vi "G5.Rest Battery Control.vi"(7 "Functions":T2, 8 "error in":errorcluster, 10 "BatteryControl_Data out":T1, 11 "G5 WEB API in":refnum<class "REST Client.lvclass">) -> (0 "error out":errorcluster, 2 "BatteryControl_Data":T1, 3 "G5 WEB API out":refnum<class "REST Client.lvclass">)   [LabVIEW 2021, in "Regatron.G5.Rest.lvlib"]
doc: "Enables using Battery Control part of G5.REST API\n- Read Energy Count\n- Read Charge Count\n- Reset Counters"
uses:
  Regatron.G5.Rest.lvlib
  <vilib>/addons/_JKI.lib/REST Client/classes/REST Client/REST Client.lvclass
  G5.Rest Battery Control Values.ctl
  G5.Rest Battery Control Functions.ctl
  Regatron.G5.Rest Handle.llb/G5.Rest JsonDB.ctl
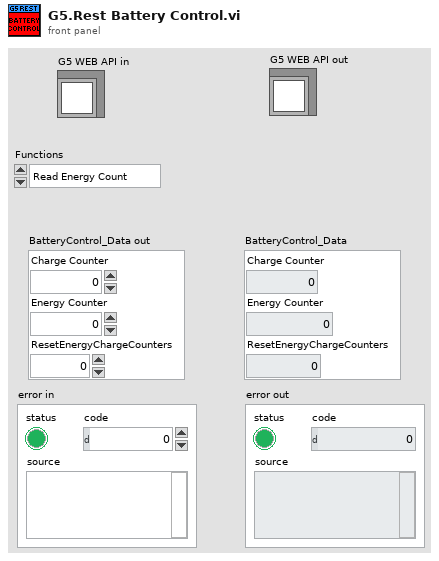
[diagram p1: front panel]
types:
  T1 = typedef "Regatron.G5.Rest.lvlib/G5.Rest Battery Control Values.ctl" = cluster{"Charge Counter":dbl, "Energy Counter":dbl, "ResetEnergyChargeCounters":dbl}
  T2 = typedef "Regatron.G5.Rest.lvlib/G5.Rest Battery Control Functions.ctl" = enum16{"Read Energy Count", "Read Charge Count", "Reset Energy Charge Counters"}
  T3 = typedef "Regatron.G5.Rest.lvlib/G5.Rest JsonDB.ctl" = cluster{"result":dbl}
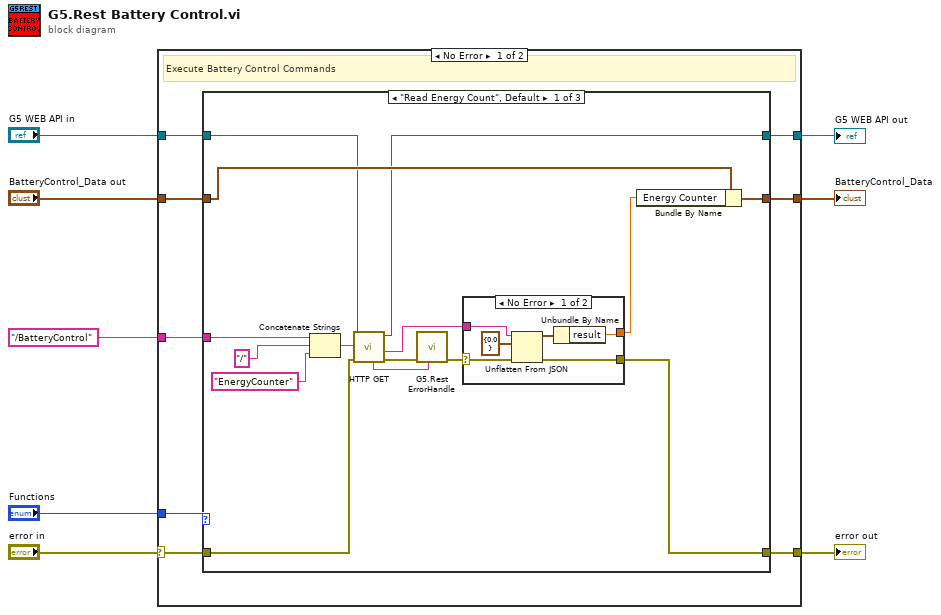
[diagram p0: block diagram]
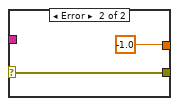
[diagram p2: hidden frame]
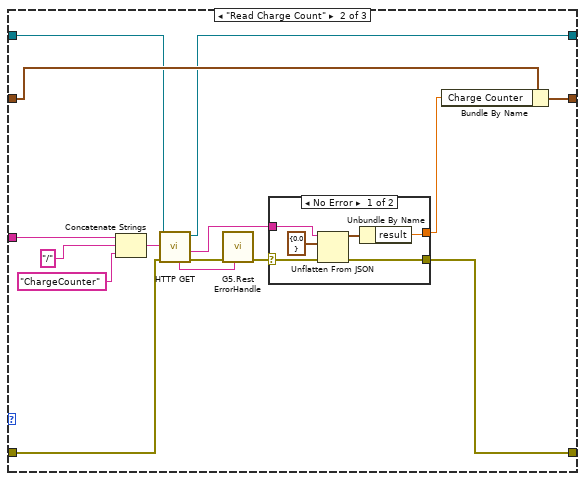
[diagram p3: hidden frame]
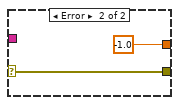
[diagram p4: hidden frame]
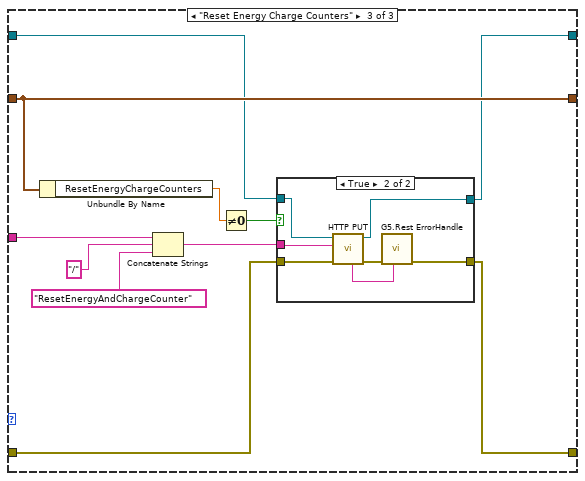
[diagram p5: hidden frame]
diagram:
  n1 = case shown="No Error" "error in" {
    selector: "error in" -> [w12 w83]
    tunnel: [w9 w85] -> w7
    tunnel: "G5 WEB API in" -> [w13 w85]
    tunnel: [w14 w84] -> w5
    tunnel: "BatteryControl_Data out" -> [w15 w84]
    tunnel: "Functions" -> [w16 _]
    tunnel: [w11 w83] -> w2
    tunnel: "/BatteryControl" ("Path") -> [w10 _]
    frame No Error {
      # "Execute Battery Control Commands"
      n2 = case shown="\"Read Energy Count\", Default" w16 {
        tunnel: w15 -> [w31 w54 w69]
        tunnel: [w30 w53 w69] -> w14
        tunnel: w13 -> [w20 w44 w65]
        tunnel: w12 -> [w17 w41 w67]
        tunnel: [w22 w46 w66] -> w11
        tunnel: w10 -> [w28 w52 w71]
        tunnel: [w18 w42 w63] -> w9
        frame "Read Energy Count", Default {
          n3 = Concatenate Strings(w28, "/" ("string"), "EnergyCounter" ("Path")) -> (w19:string)
          n4 = call-dynamic "HTTP GET.vi"("error in (no error)"=w17, "Path"=w19, "REST Client in"=w20) -> ("error out"=w25:errorcluster, "Response body"=w26:string, "REST Client out"=w18:refnum<class "REST Client.lvclass">, "Status String"=w23:string)  [unwired: 3 in, 2 out]
          n5 = call "G5.Rest ErrorHandle.vi"("Status"=w23, "error in (no error)"=w25) -> ("error out"=w24:errorcluster)  [unwired: 9 in]
          n6 = case shown="No Error" w24 {
            selector: w24 -> [w34 w39]
            tunnel: [w37 w39] -> w22
            tunnel: w26 -> [w35 _]
            tunnel: [w32 -1.0 ("result")] -> w21
            frame No Error {
              n7 = Unflatten From JSON(JSON string=w35, type and defaults=T3 {"result"=0.0} ("G5"), error in (no error)=w34) -> (value=w36:T3, error out=w37:errorcluster)  [unwired: 4 in]
              n8 = Unbundle By Name(w36) -> ("result"=w32:dbl)
            }
            frame Error {
            }
          }
          n9 = Bundle By Name(cluster=w31, "Energy Counter"=w21) -> (w30:T1)
        }
        frame "Read Charge Count" {
          n10 = Concatenate Strings(w52, "/" ("string"), "ChargeCounter" ("Path")) -> (w43:string)
          n11 = call-dynamic "HTTP GET.vi"("error in (no error)"=w41, "Path"=w43, "REST Client in"=w44) -> ("error out"=w49:errorcluster, "Response body"=w50:string, "REST Client out"=w42:refnum<class "REST Client.lvclass">, "Status String"=w47:string)  [unwired: 3 in, 2 out]
          n12 = call "G5.Rest ErrorHandle.vi"("Status"=w47, "error in (no error)"=w49) -> ("error out"=w48:errorcluster)  [unwired: 9 in]
          n13 = case shown="No Error" w48 {
            selector: w48 -> [w57 w62]
            tunnel: [w60 w62] -> w46
            tunnel: w50 -> [w58 _]
            tunnel: [w55 -1.0 ("result")] -> w45
            frame No Error {
              n14 = Unflatten From JSON(JSON string=w58, type and defaults=T3 {"result"=0.0} ("G5"), error in (no error)=w57) -> (value=w59:T3, error out=w60:errorcluster)  [unwired: 4 in]
              n15 = Unbundle By Name(w59) -> ("result"=w55:dbl)
            }
            frame Error {
            }
          }
          n16 = Bundle By Name(cluster=w54, "Charge Counter"=w45) -> (w53:T1)
        }
        frame "Reset Energy Charge Counters" {
          n17 = Unbundle By Name(w69) -> ("ResetEnergyChargeCounters"=w73:dbl)
          n18 = Concatenate Strings(w71, "/" ("string"), "ResetEnergyAndChargeCounter" ("Path")) -> (w68:string)
          n19 = Not Equal To 0?(x=w73) -> (x != 0?=w64:bool)
          n20 = case shown="True" w64 {
            tunnel: w68 -> [_ w80]
            tunnel: w67 -> [w75 w79]
            tunnel: [w75 w78] -> w66
            tunnel: w65 -> [w74 w77]
            tunnel: [w74 w76] -> w63
            frame False {
            }
            frame True {
              n21 = call-dynamic "HTTP PUT.vi"("error in (no error)"=w79, "Path"=w80, "REST Client in"=w77) -> ("error out"=w82:errorcluster, "REST Client out"=w76:refnum<class "REST Client.lvclass">, "Status String"=w81:string)  [unwired: 3 in, 3 out]
              n22 = call "G5.Rest ErrorHandle.vi"("Status"=w81, "error in (no error)"=w82) -> ("error out"=w78:errorcluster)  [unwired: 9 in]
            }
          }
        }
      }
    }
    frame Error {
      # "Pass input data in case of error"
    }
  }
  "G5 WEB API out" <- w7
  "BatteryControl_Data" <- w5
  "error out" <- w2
